vi "onCounts.vi"(2 "Value":dbl, 3 "Histogram: h(x)":u32[](array[numeric]), 4 "binning(s)":dbl) -> (0 "off times (s)":dbl[](array[numeric]), 1 "on counts":i32[](array[numeric]))   [LabVIEW 2009]
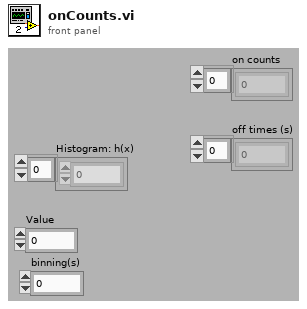
[diagram p1: front panel]
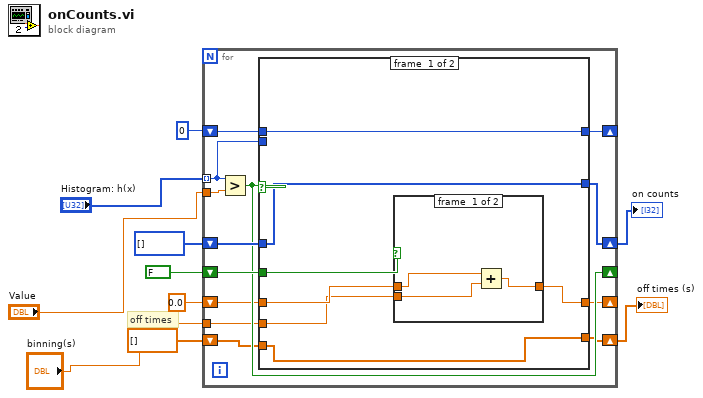
[diagram p0: block diagram]
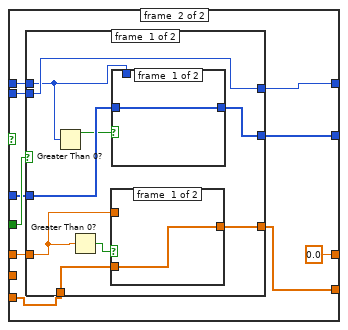
[diagram p3: hidden frame]
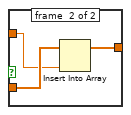
[diagram p4: hidden frame]
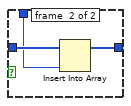
[diagram p5: hidden frame]
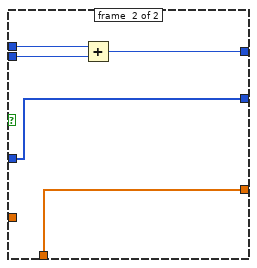
[diagram p6: hidden frame]
diagram:
  # "off times"
  n1 = for {
    tunnel: "Histogram: h(x)" -> [w21] mode=indexing
    tunnel: "Value" -> [w23]
    shift-right: [w20] -> _
    shift-left: 0 -> [w22]
    shift-right: [w16] -> _
    shift-left: FALSE -> [w19]
    shift-right: [w17] -> w10
    shift-left: i32[] [] -> [w18]
    shift-right: [w14] -> w9
    shift-left: dbl[] [] -> [w15]
    shift-right: [w12] -> _
    shift-left: 0.0 -> [w13]
    tunnel: "binning(s)" -> [w11]
    n2 = Greater?(x=w21, y=w23) -> (0:w16:bool)
    n3 = case shown="False" w16 {
      tunnel: w22 -> [w30 w44]
      tunnel: w21 -> [_ w43]
      tunnel: [w30 w42] -> w20
      tunnel: w19 -> [w28 w41]
      tunnel: w18 -> [w29 w40]
      tunnel: [w29 w39] -> w17
      tunnel: w15 -> [w25 w37]
      tunnel: [w25 w36] -> w14
      tunnel: w13 -> [w26 w38]
      tunnel: [w27 0.0 ("Value")] -> w12
      tunnel: w11 -> [w24 _]
      frame #0 {
        n4 = case shown="False" w28 {
          tunnel: [w31 w34] -> w27
          tunnel: w26 -> [w33 _]
          tunnel: w24 -> [w32 w34]
          frame #0 {
            n5 = Add(x=w33, y=w32) -> (x+y=w31:dbl)
          }
          frame #1 {
          }
        }
      }
      frame #1 {
        n6 = case shown="False" w41 {
          tunnel: w44 -> [w49 w66]
          tunnel: w43 -> [w53 w65]
          tunnel: [w53 w64] -> w42
          tunnel: w40 -> [w51 w63]
          tunnel: [w52 w63] -> w39
          tunnel: w38 -> [w47 _]
          tunnel: w37 -> [w48 w62]
          tunnel: [w45 w62] -> w36
          frame #0 {
            n7 = Greater Than 0?(x=w49) -> (x > 0?=w50:bool)
            n8 = Greater Than 0?(x=w47) -> (x > 0?=w46:bool)
            n9 = case shown="True" w46 {
              tunnel: w48 -> [w54 w57]
              tunnel: w47 -> [_ w56]
              tunnel: [w54 w55] -> w45
              frame #0 {
              }
              frame #1 {
                n10 = Insert Into Array(array=w57, new element=w56) -> (w55:dbl[])  [unwired: 1 in]
              }
            }
            n11 = case shown="True" w50 {
              tunnel: w51 -> [w58 w61]
              tunnel: w49 -> [_ w60]
              tunnel: [w58 w59] -> w52
              frame #0 {
              }
              frame #1 {
                n12 = Insert Into Array(array=w61, new element=w60) -> (w59:i32[])  [unwired: 1 in]
              }
            }
          }
          frame #1 {
            n13 = Add(x=w66, y=w65) -> (x+y=w64:u32)
          }
        }
      }
    }
  }
  "on counts" <- w10
  "off times (s)" <- w9
